vi "test_Create Instrument Addon from Config.vi"(8 "error in (no error)":errorcluster, 11 "TestCase in":refnum<class "Instrument Addon Scripting API Custom Device Unit Tests.lvclass">) -> (0 "error out":errorcluster, 3 "TestCase out":refnum<class "Instrument Addon Scripting API Custom Device Unit Tests.lvclass">)   [LabVIEW 2019, in "Instrument Addon Scripting API Custom Device Unit Tests.lvclass"]
uses:
  Instrument Addon Scripting API Custom Device Unit Tests.lvclass
  Instrument Addon Scripting API Custom Device Unit Tests.lvclass/Instrument Addon Scripting API Custom Device Unit Tests.ctl
  <vilib>/addons/_JKI Toolkits/VI Tester/TestCase.llb/TestCase.lvclass
  Instrument Addon Scripting API Test Assets/Instrument Addon Scripting API Test Assets.lvclass
  APIs/Scripting API/Instrument Addon Scripting API.lvlib
  C:/Program Files (x86)/National Instruments/LabVIEW 2019/vi.lib/addons/_JKI Toolkits/VI Tester/TestCase.llb/TestCase.lvclass
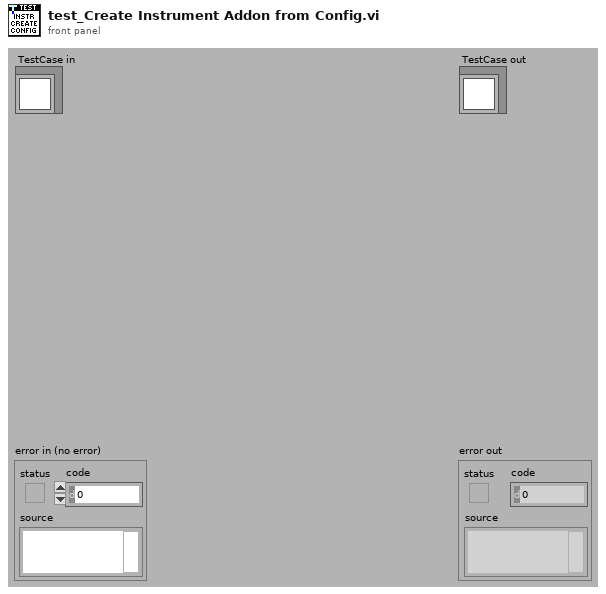
[diagram p1: front panel]
types:
  T1 = typedef "Custom Device API.lvlib/Custom Device Item Ref.ctl" = u64
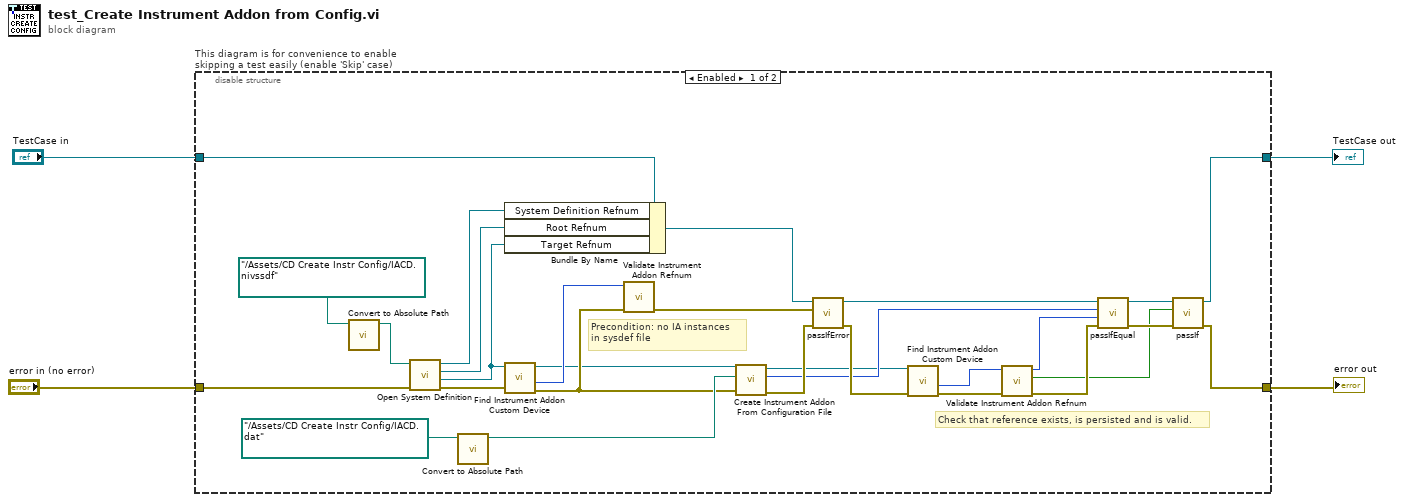
[diagram p0: block diagram]
diagram:
  n1 = disable-structure "This diagram is for convenience to enable skipping a test easily (enable 'Skip' case)" shown="Enabled" {
    disable-tunnel: "TestCase in" -> [w29 w37]
    disable-tunnel: [w8 w35] -> w1
    disable-tunnel: [w10 w36] -> w3
    disable-tunnel: "error in (no error)" -> [w33 w34]
    frame Enabled {
      # "Check that reference exists, is persisted and is valid."
      # "Precondition: no IA instances\nin sysdef file"
      n2 = call "Convert to Absolute Path.vi"("System Definition File"=path "../Assets/CD Create Instr Config/IACD.nivssdf" ("SDF file")) -> ("Absolute Path"=w31:path)  [unwired: 10 in]
      n3 = call "Open System Definition.vi"("error in (no error)"=w33, "System Definition File"=w31) -> ("error out"=w25:errorcluster, "Target Refnum"=w24:refnum<k24>, "Root Refnum"=w27:refnum<k24>, "System Definition Refnum"=w28:refnum<k24>)  [unwired: 6 in]
      n4 = call "Convert to Absolute Path.vi"("System Definition File"=path "../Assets/CD Create Instr Config/IACD.dat" ("SDF file")) -> ("Absolute Path"=w26:path)  [unwired: 10 in]
      n5 = Bundle By Name(cluster=w29, "System Definition Refnum"=w28, "Root Refnum"=w27, "Target Refnum"=w24) -> (w19:refnum<class "Instrument Addon Scripting API Custom Device Unit Tests.lvclass">)
      n6 = call "Find Instrument Addon Custom Device.vi"("error in"=w25, "target in"=w24) -> ("error out"=w21:errorcluster, "NodeID"=w23:u64, "target out"=w6:refnum<k24>)  [unwired: 7 in]
      n7 = call "Validate Instrument Addon Refnum.vi"("Error In"=w21, "Refnum In"=w23) -> ("Error Out"=w20:errorcluster)  [unwired: 7 in, 2 out]
      n8 = call "Create Instrument Addon From Configuration File.vi"("error in (no error)"=w21, "configuration file path"=w26, "target in"=w6) -> ("error out"=w22:errorcluster, "instrument addon refnum"=w12:T1, "target out"=w5:refnum<k24>)  [unwired: 6 in]
      n9 = call-dynamic "passIfError.vi"("error in (no error)"=w22, "error"=w20, "TestCase in"=w19) -> ("error out"=w17:errorcluster, "TestCase out"=w15:refnum<class "Instrument Addon Scripting API Custom Device Unit Tests.lvclass">)  [unwired: 7 in]
      n10 = call "Find Instrument Addon Custom Device.vi"("error in"=w17, "target in"=w5) -> ("error out"=w16:errorcluster, "NodeID"=w18:u64)  [unwired: 7 in, 1 out]
      n11 = call "Validate Instrument Addon Refnum.vi"("Error In"=w16, "Refnum In"=w18) -> ("Error Out"=w14:errorcluster, "Is Instrument Addon?"=w7:bool, "Refnum Out"=w13:T1)  [unwired: 7 in]
      n12 = call-dynamic "passIfEqual.vi"("error in (no error)"=w14, "y"=w13, "x"=w12, "TestCase in"=w15) -> ("error out"=w11:errorcluster, "TestCase out"=w9:refnum<class "Instrument Addon Scripting API Custom Device Unit Tests.lvclass">)  [unwired: 6 in]
      n13 = call-dynamic "passIf.vi"("error in (no error)"=w11, "pass"=w7, "TestCase in"=w9) -> ("error out"=w10:errorcluster, "TestCase out"=w8:refnum<class "Instrument Addon Scripting API Custom Device Unit Tests.lvclass">)  [unwired: 7 in]
    }
    frame Disabled {
      # "skip test result while test is under development"
      n14 = call <vilib>:"skip.vi"("error in (no error)"=w34, "TestCase in"=w37) -> ("error out"=w36:errorcluster, "TestCase out"=w35:refnum<class "Instrument Addon Scripting API Custom Device Unit Tests.lvclass">)  [unwired: 8 in]
    }
  }
  "error out" <- w3
  "TestCase out" <- w1
